vi "Get Firmware Version.vi"(8 "error in (no error)":errorcluster) -> (0 "error out":errorcluster, 3 "Firmware Version String":string)   [LabVIEW 2015, in "Tool Interface.lvlib"]
uses:
  Tool Interface.lvlib
panel:
  out "Message":string
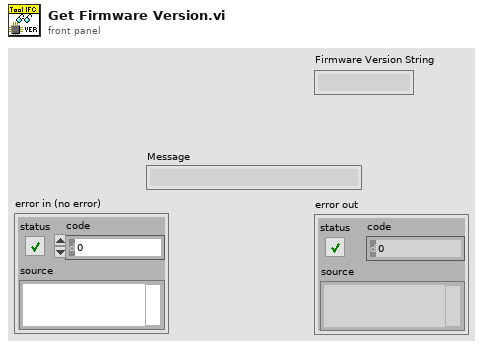
[diagram p1: front panel]
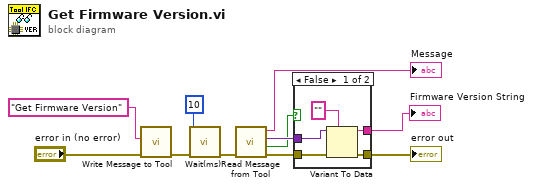
[diagram p0: block diagram]
diagram:
  n1 = call "Write Message to Tool.vi"("error in (no error)"="error in (no error)", "Message"="Get Firmware Version") -> ("error out"=w9:errorcluster)  [unwired: 9 in]
  n2 = call "Wait(ms).vi"("error in (no error)"=w9, "milliseconds"=u32 10) -> ("error out"=w8:errorcluster)  [unwired: 9 in]
  n3 = call "Read Message from Tool.vi"("error in (no error)"=w8) -> ("error out"=w5:errorcluster, "timed out?"=w2:bool, "Message Data"=w6:variant, "Message"=→"Message":string)  [unwired: 7 in]
  n4 = case shown="False" w2 {
    tunnel: w6 -> [w16 _]
    tunnel: w5 -> [w15 w17]
    tunnel: [w14 _] -> w4
    tunnel: [w12 w17] -> w3
    frame False {
      n5 = Variant To Data(error in=w15, type="", Variant=w16) -> (data=w14:string, error out=w12:errorcluster)
    }
    frame True {
    }
  }
  "error out" <- w3
  "Firmware Version String" <- w4
